vi "Pre Launch Init.vi"(11 "Analog Input in":refnum<class "Analog Input.lvclass">) -> (0 "error out":errorcluster, 3 "Analog Input out":refnum<class "Analog Input.lvclass">)   [LabVIEW 2021, in "Analog Input.lvlib" / "Analog Input.lvclass"]
doc: "(<B>Filename</B>: Actor Framework.lvlib:Actor.lvclass:Pre Launch Init.vi)\n\nDefines behavior that occurs after the Launch Nested Actor method is invoked but before the actor's Actor Core method begins running.\n\nBy default, this method does nothing. A descendant class may override it to define behavior."
uses:
  Analog Input.lvclass
  C:/Program Files/National Instruments/LabVIEW 2021/vi.lib/ActorFramework/Actor/Actor.lvclass
  Analog Input.lvclass/Analog Input.ctl
  <vilib>/ActorFramework/Actor/Actor.lvclass/Actor.ctl
  <vilib>/ActorFramework/Message Enqueuer/Message Enqueuer.lvclass/Message Enqueuer.ctl
  <vilib>/ActorFramework/Message Enqueuer/Enqueue.vi
  <vilib>/ActorFramework/Message Enqueuer/Init from Existing Queue.vi
  Analog Input Messages/Acquire Voltage Msg/Acquire Voltage Msg.lvclass
  C:/Program Files/National Instruments/LabVIEW 2021/vi.lib/ActorFramework/Message/Message.lvclass
  <vilib>/DAQmx/configure/timing.llb/DAQmx Timing (Sample Clock).vi
  <vilib>/ActorFramework/Message Priority Queue/Priority Enqueue.vi
  <vilib>/ActorFramework/Actor/Actor.lvclass
  <vilib>/ActorFramework/Message Enqueuer/Message Enqueuer.lvclass
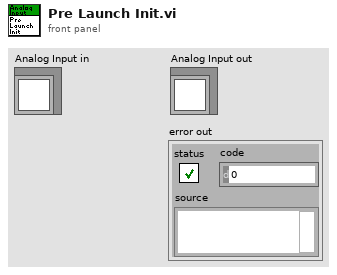
[diagram p1: front panel]
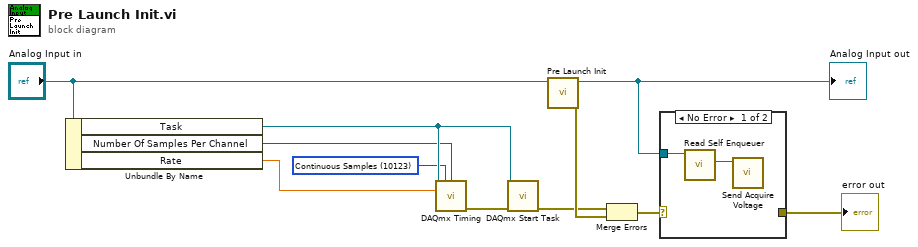
[diagram p0: block diagram]
diagram:
  w1 = 10123 items=["Finite Samples"=10178, "Continuous Samples"=10123, "Hardware Timed Single Point"=12522] ("sample mode")
  n1 = Unbundle By Name("Analog Input in") -> ("Task"=w6:refnum<k21>, "Number Of Samples Per Channel"=w5:i32, "Rate"=w10:dbl)
  n2 = call-poly <vilib>:"DAQmx Timing.vi"("task/channels in"=w6, "sample mode"=w1, "samples per channel"=w5, "rate"=w10) -> ("error out"=w8:errorcluster)  [unwired: 10 in, 1 out]
  n3 = call <vilib>:"DAQmx Start Task.vi"("task/channels in"=w6, "error in"=w8) -> ("error out"=w9:errorcluster)  [unwired: 12 in, 1 out]
  n4 = call-parent "Pre Launch Init.vi"("Actor in"="Analog Input in") -> ("error out"=w11:errorcluster, "Actor out"=w2:refnum<class "Analog Input.lvclass">)  [unwired: 9 in]
  "Analog Input out" <- w2
  n5 = Merge Errors(w9, w11) -> (w4:errorcluster)
  n6 = case shown="No Error" w4 {
    selector: w4 -> [_ w14]
    tunnel: w2 -> [w12 _]
    tunnel: [_ w14] -> w3
    frame No Error {
      n7 = call <vilib>:"Read Self Enqueuer.vi"("Actor"=w12) -> ("Self Enqueuer"=w13:refnum<class "Message Enqueuer.lvclass">)  [unwired: 10 in]
      n8 = call "Send Acquire Voltage.vi"("Message Enqueuer"=w13) -> ()  [unwired: 9 in, 2 out]
    }
    frame Error {
    }
  }
  "error out" <- w3
